vi "Multiplot_graph.vi"() -> ()   [LabVIEW 2012]
panel:
  in  "?":bool
  in  "SquareWave \nFrequency":dbl(slide) scale=0.0..10.0
  in  "Sinewave \nFrequency":dbl(slide) scale=0.0..10.0
  out "Waveform Graph":dynamicdata(graph)
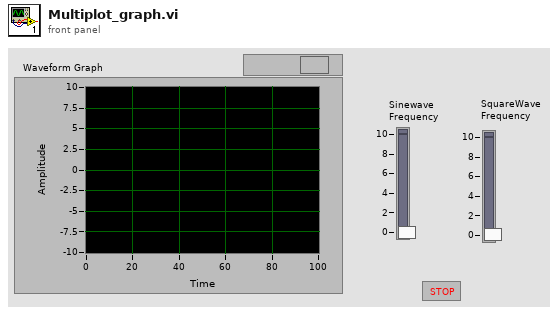
[diagram p1: front panel]
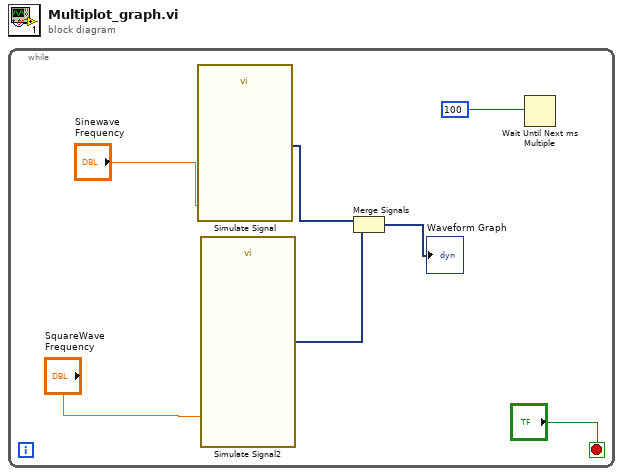
[diagram p0: block diagram]
diagram:
  n1 = while {
    stop <- "?" stop-if-true
    n2 = call "Simulate Signal"("Frequency"="Sinewave \nFrequency") -> ("Sine"=w5:dynamicdata)  [unwired: 13 in, 1 out]
    n3 = call "Simulate Signal2"("Frequency"="SquareWave \nFrequency") -> ("Square"=w4:dynamicdata)  [unwired: 13 in, 1 out]
    n4 = Merge Signals(w5, w4) -> (→"Waveform Graph":dynamicdata)
    n5 = Wait Until Next ms Multiple(millisecond multiple=100) -> ()  [unwired: 1 out]
  }
